vi "Init Series.vi"(6 "Series CFG":string, 8 "error in":errorcluster, 9 "Virt Instrs CFG":string, 10 "Instr CFGs":string[](array[string]), 11 "Host MSS Test Actor in":refnum<class "Host MSS Test Actor.lvclass">) -> (0 "error out":errorcluster, 3 "Host MSS Test Actor out":refnum<class "Host MSS Test Actor.lvclass">)   [LabVIEW 2023, in "Host MSS Test Actor.lvlib" / "Host MSS Test Actor.lvclass"]
uses:
  Host MSS Test Actor.lvclass
  C:/Program Files/National Instruments/LabVIEW 2023/vi.lib/ActorFramework/Actor/Actor.lvclass
  Task/Task Actor/Task Actor/Task Actor/Task Actor.lvclass
  <vilib>/ActorFramework/Message Enqueuer/Message Enqueuer.lvclass
  Host MSS Test Actor.lvclass/Host MSS Test Actor.ctl
  Series/Series Base/Series Base.lvclass/Series Base.ctl
  Task/Task Actor/Task Actor/Task Actor/Task Actor.lvclass/Task Actor.ctl
  Series/Series Base/Series Base.lvclass
  <vilib>/ActorFramework/Actor/Actor.lvclass
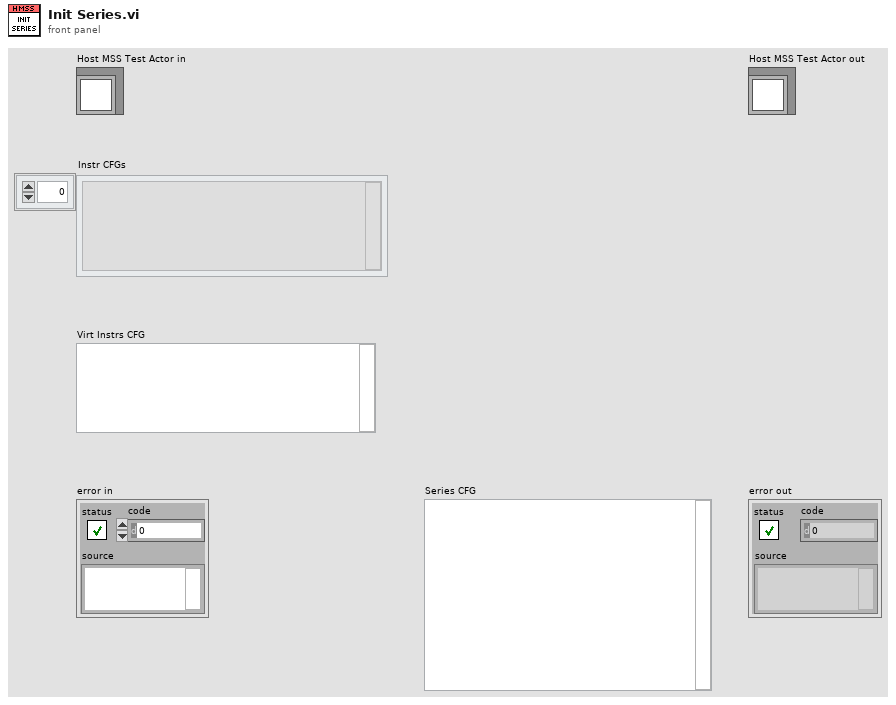
[diagram p1: front panel]
types:
  T1 = map{string, refnum<class "Message Enqueuer.lvclass">}
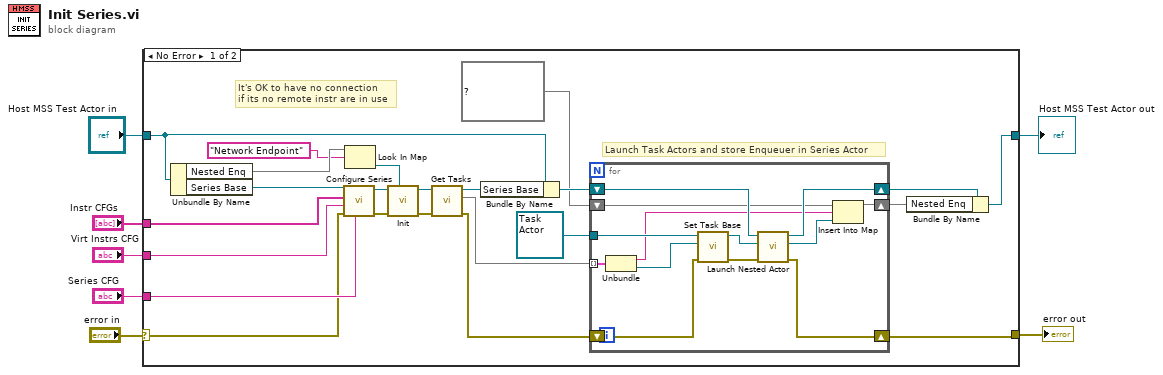
[diagram p0: block diagram]
diagram:
  n1 = case shown="No Error" "error in" {
    selector: "error in" -> [w12 w45]
    tunnel: [w15 w45] -> w6
    tunnel: [w14 w44] -> w4
    tunnel: "Host MSS Test Actor in" -> [w19 w44]
    tunnel: "Instr CFGs" -> [w29 _]
    tunnel: "Virt Instrs CFG" -> [w28 _]
    tunnel: "Series CFG" -> [w27 _]
    frame No Error {
      # "It's OK to have no connection\nif its no remote instr are in use"
      # "Launch Task Actors and store Enqueuer in Series Actor"
      n2 = Unbundle By Name(w19) -> ("Nested Enq"=w10:T1, "Series Base"=w30:refnum<class "Series Base.lvclass">)
      n3 = call "Configure Series.vi"("Series CFG"=w27, "error in (no error)"=w12, "Virt Instrs CFG"=w28, "Instr CFGs"=w29, "HAL GOOP4:Series Base in"=w30) -> ("error out"=w26:errorcluster, "HAL GOOP4:Series Base out"=w24:refnum<class "Series Base.lvclass">)  [unwired: 5 in]
      n4 = Look In Map(map=w10, key="Network Endpoint") -> (value=w8:refnum<class "Message Enqueuer.lvclass">)  [unwired: 1 in, 1 out]
      n5 = call-dynamic "Init.vi"("Target Enqueuer"=w8, "error in (no error)"=w26, "HAL GOOP4:Series Base in"=w24) -> ("error out"=w25:errorcluster, "HAL GOOP4:Series Base out"=w23:refnum<class "Series Base.lvclass">)  [unwired: 7 in]
      n6 = call "Get Tasks.vi"("error in (no error)"=w25, "HAL GOOP4:Series Base in"=w23) -> ("error out"=w16:errorcluster, "Tasks"=w21:map{string, refnum<class "Task Base.lvclass">}, "HAL GOOP4:Series Base out"=w22:refnum<class "Series Base.lvclass">)  [unwired: 7 in]
      n7 = Bundle By Name(cluster=w19, "Series Base"=w22) -> (w18:refnum<class "Host MSS Test Actor.lvclass">)
      n8 = for {
        tunnel: w21 -> [w33] mode=indexing
        shift-right: [w37] -> w17
        shift-left: w18 -> [w43]
        tunnel: refnum<class "Task Actor.lvclass"> refnum ("Task Actor.lvlib:Task Actor.lvclass") -> [w42]
        shift-right: [w38] -> w15
        shift-left: w16 -> [w40]
        shift-right: [w35] -> w13
        shift-left: T1 {} ("Size: 0") -> [w36]
        n9 = Unbundle(w33) -> (w32:string, "Task"=w31:refnum<class "Task Base.lvclass">)
        n10 = call "Set Task Base.vi"("error in (no error)"=w40, "HAL GOOP4.lvlib:Task Base.lvclass"=w31, "Task Actor in"=w42) -> ("error out"=w39:errorcluster, "Task Actor out"=w41:refnum<class "Task Actor.lvclass">)  [unwired: 7 in]
        n11 = call <vilib>:"Launch Nested Actor.vi"("error in (no error)"=w39, "Nested Actor"=w41, "Caller Actor in"=w43) -> ("error out"=w38:errorcluster, "Nested Actor's Enqueuer"=w34:refnum<class "Message Enqueuer.lvclass">, "Caller Actor out"=w37:refnum<class "Host MSS Test Actor.lvclass">)  [unwired: 6 in]
        n12 = Insert Into Map(map in=w36, key=w32, value=w34) -> (map out=w35:T1)  [unwired: 2 out]
      }
      n13 = Bundle By Name(cluster=w17, "Nested Enq"=w13) -> (w14:refnum<class "Host MSS Test Actor.lvclass">)
    }
    frame Error {
    }
  }
  "error out" <- w6
  "Host MSS Test Actor out" <- w4
